vi "DumbDash Load Controls.vi"(11 "TabControl in":refnum<vi>) -> (3 "Array":T1[](array[typedef]))   [LabVIEW 2015]
uses:
  DumbDash Control.ctl
  DumbDash Control Type.ctl
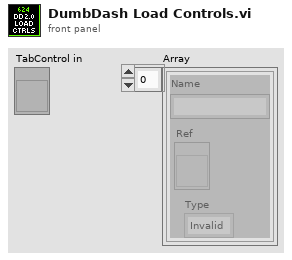
[diagram p1: front panel]
types:
  T1 = typedef "DumbDash Control.ctl" = cluster{"Name":string, "Ref":refnum<vi>, "Type":T2}
  T2 = typedef "DumbDash Control Type.ctl" = enum16{"Invalid", "Number", "Boolean", "String"}
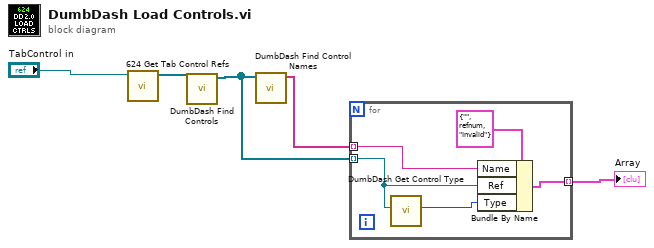
[diagram p0: block diagram]
diagram:
  n1 = call "624 Get Tab Control Refs.vi"("TabControl in"="TabControl in") -> ("ControlsOnPage"=w2:refnum<vi>[])  [unwired: 10 in]
  n2 = call "DumbDash Find Controls.vi"("ControlsOnPage"=w2) -> ("Found Controls"=w3:refnum<vi>[])  [unwired: 10 in]
  n3 = call "DumbDash Find Control Names.vi"("Controls"=w3) -> ("Dashboard Names"=w4:string[])  [unwired: 10 in]
  n4 = for {
    tunnel: w3 -> [w8] mode=indexing
    tunnel: w4 -> [w9] mode=indexing
    tunnel: [w6] -> w5 mode=indexing
    n5 = call "DumbDash Get Control Type.vi"("reference"=w8) -> ("Type"=w7:T2)  [unwired: 10 in]
    n6 = Bundle By Name(cluster=T1 {"Name"="", "Ref"=refnum, "Type"=enum."Invalid"} ("Cluster"), "Name"=w9, "Ref"=w8, "Type"=w7) -> (w6:T1)
  }
  "Array" <- w5
